vi "Drag Leave.vi"(8 "error in (no error)":errorcluster, 11 "BetterHandle in":refnum<class "BetterHandle.lvclass">) -> (0 "error out":errorcluster, 3 "BetterHandle out":refnum<class "BetterHandle.lvclass">)   [LabVIEW 2020, in "BetterDragAndDrop.lvlib" / "BetterHandle.lvclass"]
uses:
  BetterHandle.lvclass
  BetterHandle.lvclass/BetterHandle.ctl
  BetterTreeBar/SubVIs/Horizontal Bar Enumeration.ctl
  BetterTreeBar/BetterHorizontalBar.lvclass
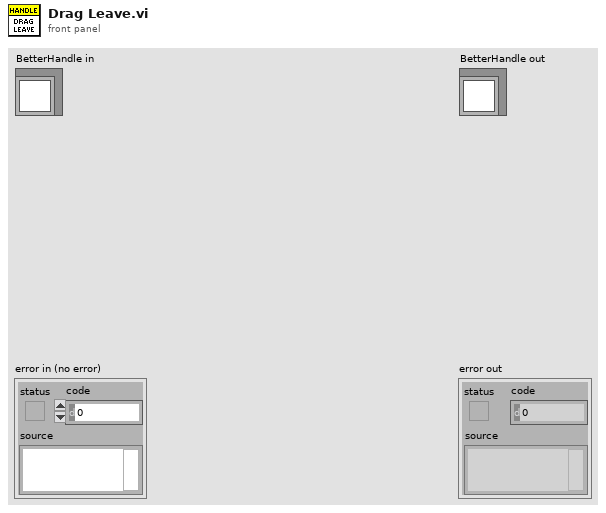
[diagram p1: front panel]
types:
  T1 = typedef "BetterDragAndDrop.lvlib/BetterHorizontalBar.lvclass/Horizontal Bar Enumeration.ctl" = enum16{"None", "only bar", "tilda up"}
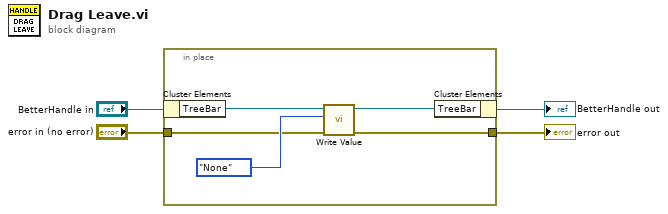
[diagram p0: block diagram]
diagram:
  n1 = in-place {
    in-place-border: [w5] -> w1
    in-place-border: "error in (no error)" -> [w6]
    n2 = in-place-cluster #1("BetterHandle in") -> ("TreeBar"=w9:refnum<class "BetterHorizontalBar.lvclass">)
    n3 = call "Write Value.vi"("error in (no error)"=w6, "New Value"=Horizontal_Bar_Enumeration."None", "BetterTreeBar in"=w9) -> ("error out"=w5:errorcluster, "BetterTreeBar out"=w8:refnum<class "BetterHorizontalBar.lvclass">)  [unwired: 7 in]
    n4 = in-place-cluster #1("TreeBar"=w8) -> (→"BetterHandle out":refnum<class "BetterHandle.lvclass">)
  }
  "error out" <- w1
